vi "Handle Command.vi"(8 "error in (no error)":errorcluster, 9 "Data":variant, 10 "Command":string, 11 "instrument.PPMS2 in":refnum<class "instrument.PPMS.lvclass">) -> (0 "error out":errorcluster, 1 "Processed Data":variant, 2 "Command":string, 3 "instrument.PPMS2 out":refnum<class "instrument.PPMS.lvclass">)   [LabVIEW 2016, in "instrument.PPMS.lvclass"]
uses:
  instrument.PPMS.lvclass
  Typedefs/Temperature--PPMS--cluster.ctl
  instrument.PPMS.lvclass/instrument.PPMS.ctl
  Typedefs/Magnet Field--PPMS--cluster.ctl
  <userlib>/LevyLab/Levylab Instruments/Instrument Types/Cryostat/Typedefs/Magnet Mode--Enum.ctl
  Typedefs/Magnet Status--PPMS--cluster.ctl
  Typedefs/Magnet Status--PPMS--ring.ctl
  Typedefs/Temperature Status--PPMS--cluster.ctl
  <userlib>/LevyLab/Levylab Instruments/Instrument Types/Cryostat/Instrument.Cryostat.lvclass
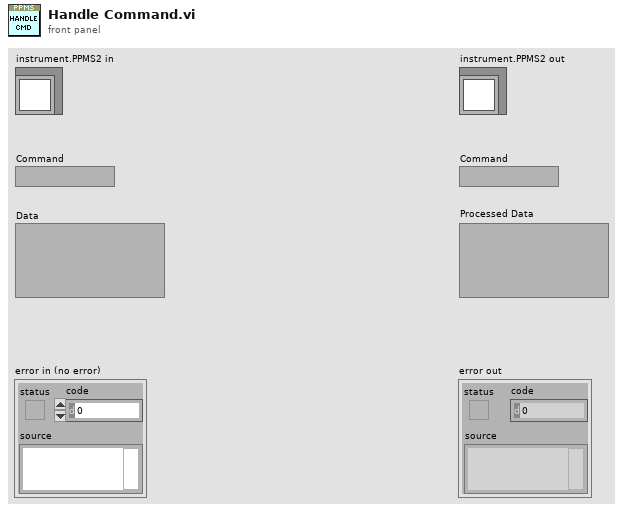
[diagram p1: front panel]
types:
  T1 = typedef "instrument.PPMS.lvclass/Temperature--PPMS--cluster.ctl" = cluster{"Temperature (K)":dbl, "Rate (K/min)":dbl}
  T2 = typedef "instrument.PPMS.lvclass/Magnet Field--PPMS--cluster.ctl" = cluster{"Target Field (Oe)":dbl, "Target Rate (Oe/s)":dbl, "Mode":T3}
  T3 = typedef "Instrument.Cryostat.lvclass/Magnet Mode--Enum.ctl" = enum16{"Persistent", "Driven"}
  T4 = typedef "instrument.PPMS.lvclass/Magnet Status--PPMS--cluster.ctl" = cluster{"Field (Oe)":dbl, "Field Status":T5}
  T5 = typedef "instrument.PPMS.lvclass/Magnet Status--PPMS--ring.ctl" = i32
  T6 = typedef "instrument.PPMS.lvclass/Temperature Status--PPMS--cluster.ctl" = cluster{"Temperature (K)":dbl, "Temperature Status":i32}
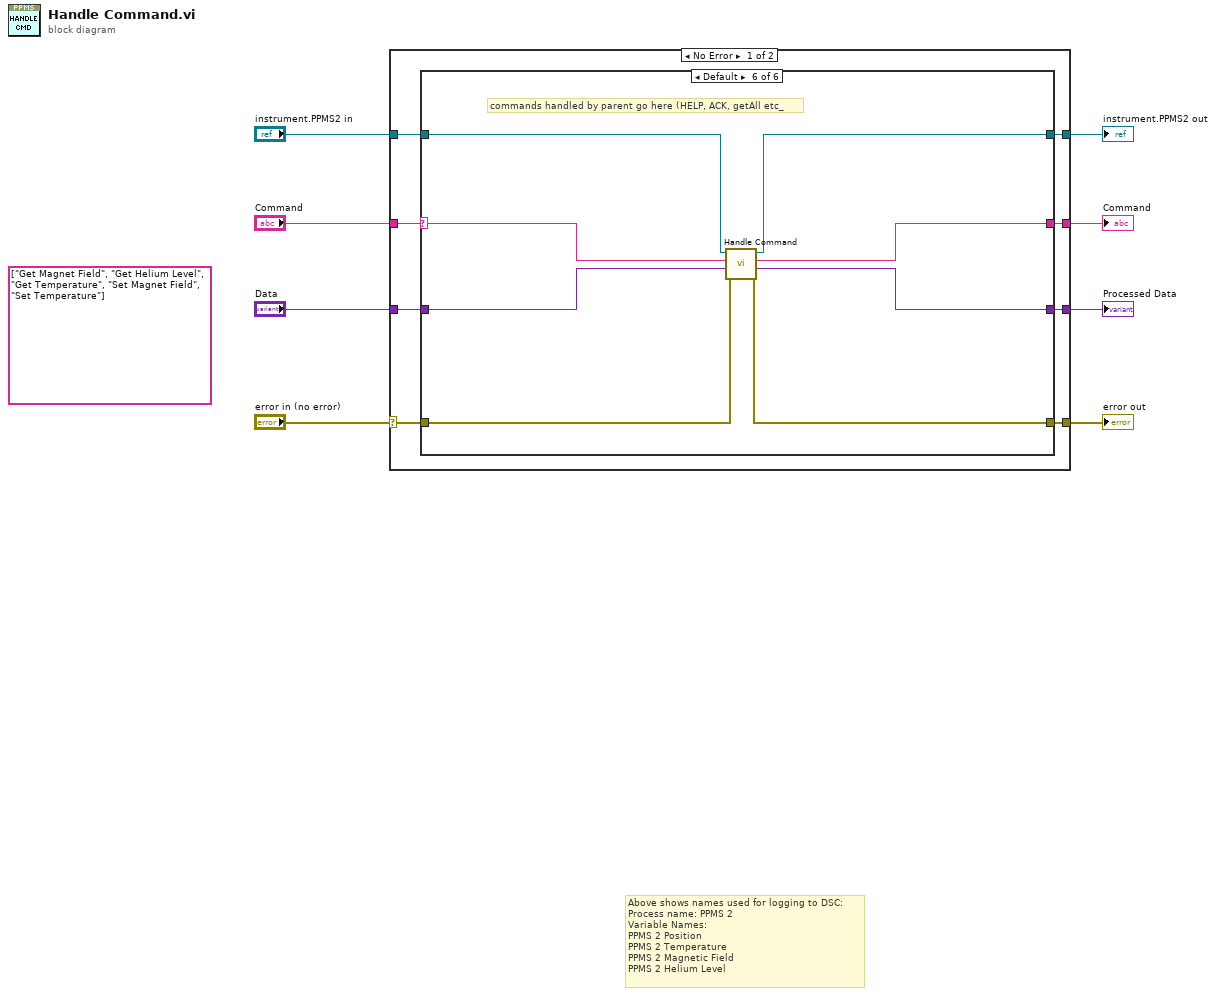
[diagram p0: block diagram]
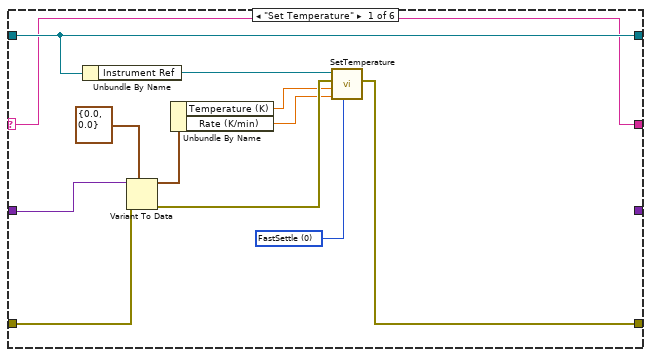
[diagram p2: hidden frame]
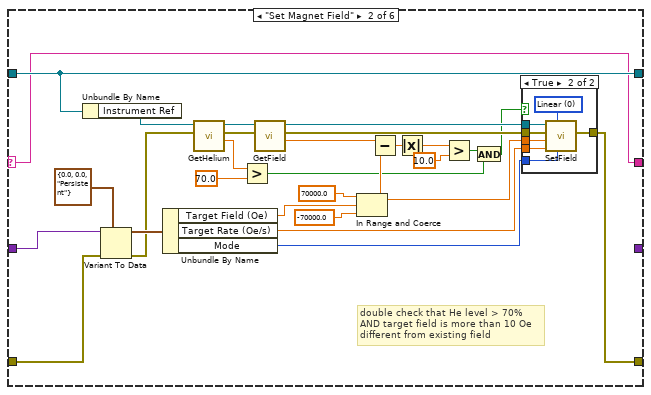
[diagram p3: hidden frame]
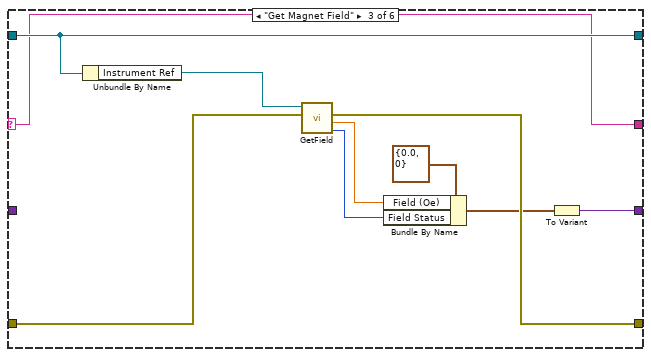
[diagram p5: hidden frame]
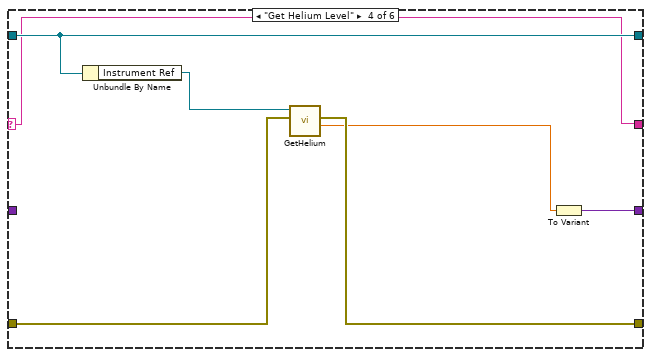
[diagram p6: hidden frame]
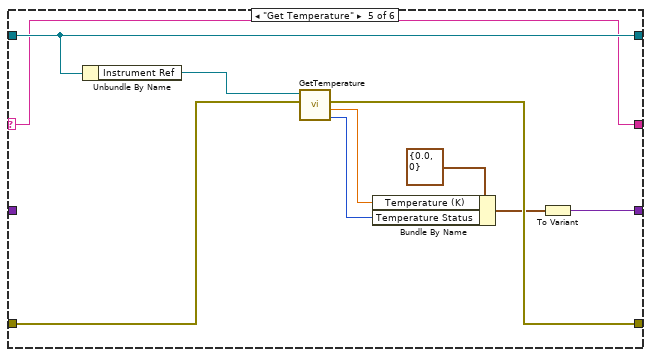
[diagram p7: hidden frame]
diagram:
  (unwired) string[] ["Get Magnet Field", "Get Helium Level", "Get Temperature", "Set Magnet Field", "Set Temperature"] ("Commands")
  # "Above shows names used for logging to DSC:\nProcess name: PPMS 2\nVariable Names:\nPPMS 2 Position\nPPMS 2 Temperature\nPPMS 2 Magnetic Field\nPPMS 2 Helium Level"
  n1 = case shown="No Error" "error in (no error)" {
    selector: "error in (no error)" -> [w11 w100]
    tunnel: [w10 w100] -> w6
    tunnel: [w16 _] -> w4
    tunnel: [w15 _] -> w5
    tunnel: [w14 w101] -> w7
    tunnel: "Data" -> [w13 _]
    tunnel: "Command" -> [w9 _]
    tunnel: "instrument.PPMS2 in" -> [w12 w101]
    frame No Error {
      n2 = case shown="Default" w9 {
        selector: w9 -> [w17 w29 w65 w75 w82 w92]
        tunnel: [_ _ w66 w77 w87 w99] -> w16
        tunnel: [w17 w29 w65 w75 w82 w98] -> w15
        tunnel: [w28 w56 w74 w81 w91 w97] -> w14
        tunnel: w13 -> [w23 w54 _ _ _ w96]
        tunnel: w12 -> [w28 w56 w74 w81 w91 w95]
        tunnel: w11 -> [w25 w53 w72 w80 w89 w94]
        tunnel: [w26 w51 w71 w79 w88 w93] -> w10
        frame "Set Temperature" {
          w18 = 0 items=["FastSettle", "NoOvershoot"] ("Approach")
          n3 = Unbundle By Name(w28) -> ("Instrument Ref"=w27:refnum<k24>)
          n4 = Variant To Data(error in=w25, type=T1 {"Temperature (K)"=0.0, "Rate (K/min)"=0.0} ("Temperature"), Variant=w23) -> (data=w22:T1, error out=w21:errorcluster)
          n5 = Unbundle By Name(w22) -> ("Temperature (K)"=w20:dbl, "Rate (K/min)"=w19:dbl)
          n6 = call "SetTemperature.vi"("Approach"=w18, "Rate"=w19, "Temperature"=w20, "error in (no error)"=w21, "Instrument Ref In"=w27) -> ("error out"=w26:errorcluster)  [unwired: 2 in, 2 out]
        }
        frame "Set Magnet Field" {
          # "double check that He level > 70%\nAND target field is more than 10 Oe\ndifferent from existing field"
          n7 = Unbundle By Name(w56) -> ("Instrument Ref"=w37:refnum<k24>)
          n8 = Variant To Data(error in=w53, type=T2 {"Target Field (Oe)"=0.0, "Target Rate (Oe/s)"=0.0, "Mode"=enum."Persistent"} ("Magnet Field"), Variant=w54) -> (data=w52:T2, error out=w50:errorcluster)
          n9 = Unbundle By Name(w52) -> ("Target Field (Oe)"=w40:dbl, "Target Rate (Oe/s)"=w43:dbl, "Mode"=w31:T3)
          n10 = call "GetHelium.vi"("error in (no error)"=w50, "Instrument Refnum in"=w37) -> ("Helium Level (%)"=w44:dbl, "error out"=w49:errorcluster, "Instrument Ref Out"=w47:refnum<k24>)  [unwired: 3 in]
          n11 = Greater?(x=w44, y=70.0) -> (0:w32:bool)
          n12 = call "GetField.vi"("error in (no error)"=w49, "Instrument Ref In"=w47) -> ("Field"=w35:dbl, "error out"=w48:errorcluster, "Instrument Ref Out"=w46:refnum<k24>)  [unwired: 3 in, 2 out]
          n13 = In Range and Coerce(upper limit=70000.0, x=w40, lower limit=-70000.0) -> (coerced(x)=w36:dbl)  [unwired: 1 out]
          n14 = Subtract(x=w35, y=w36) -> (x-y=w34:dbl)
          n15 = Absolute Value(x=w34) -> (abs(x)=w39:dbl)
          n16 = Greater?(x=w39, y=10.0) -> (0:w33:bool)
          n17 = And(x=w33, y=w32) -> (x .and. y?=w30:bool)
          n18 = case shown="True" w30 {
            tunnel: [w57 w63] -> w51
            tunnel: w48 -> [w57 w62]
            tunnel: w46 -> [_ w61]
            tunnel: w43 -> [_ w60]
            tunnel: w36 -> [_ w59]
            tunnel: w31 -> [_ w58]
            frame False {
            }
            frame True {
              w64 = 0 items=["Linear", "NoOvershoot", "Oscillate"] ("Approach")
              n19 = call "SetField.vi"("Mode"=w58, "Approach"=w64, "Rate"=w60, "Field"=w59, "error in (no error)"=w62, "Instrument Ref In"=w61) -> ("error out"=w63:errorcluster)  [unwired: 1 in, 2 out]
            }
          }
        }
        frame "Get Magnet Field" {
          n20 = Unbundle By Name(w74) -> ("Instrument Ref"=w73:refnum<k24>)
          n21 = call "GetField.vi"("error in (no error)"=w72, "Instrument Ref In"=w73) -> ("Field\nStatus"=w69:i32, "Field"=w70:dbl, "error out"=w71:errorcluster)  [unwired: 3 in, 2 out]
          n22 = Bundle By Name(cluster=T4 {"Field (Oe)"=0.0, "Field Status"=0}, "Field (Oe)"=w70, "Field Status"=w69) -> (w67:T4)
          n23 = To Variant(anything=w67) -> (Variant=w66:variant)
        }
        frame "Get Helium Level" {
          n24 = Unbundle By Name(w81) -> ("Instrument Ref"=w76:refnum<k24>)
          n25 = call "GetHelium.vi"("error in (no error)"=w80, "Instrument Refnum in"=w76) -> ("Helium Level (%)"=w78:dbl, "error out"=w79:errorcluster)  [unwired: 3 in, 1 out]
          n26 = To Variant(anything=w78) -> (Variant=w77:variant)
        }
        frame "Get Temperature" {
          n27 = Unbundle By Name(w91) -> ("Instrument Ref"=w90:refnum<k24>)
          n28 = call "GetTemperature.vi"("error in (no error)"=w89, "Instrument Ref In"=w90) -> ("Temperature\nStatus"=w85:i32, "Temperature"=w86:dbl, "error out"=w88:errorcluster)  [unwired: 3 in, 2 out]
          n29 = Bundle By Name(cluster=T6 {"Temperature (K)"=0.0, "Temperature Status"=0}, "Temperature (K)"=w86, "Temperature Status"=w85) -> (w83:T6)
          n30 = To Variant(anything=w83) -> (Variant=w87:variant)
        }
        frame Default {
          # "commands handled by parent go here (HELP, ACK, getAll etc_"
          n31 = call-parent "Handle Command.vi"("error in (no error)"=w94, "Data"=w96, "Command"=w92, "Instrument in"=w95) -> ("error out"=w93:errorcluster, "Processed Data"=w99:variant, "Command"=w98:string, "Instrument out"=w97:refnum<class "instrument.PPMS.lvclass">)  [unwired: 4 in]
        }
      }
    }
    frame Error {
    }
  }
  "error out" <- w6
  "instrument.PPMS2 out" <- w7
  "Processed Data" <- w4
  "Command" <- w5
